vi "Obtain Queue Registry.vi"(8 "error in (no error)":errorcluster) -> (0 "error out":errorcluster, 2 "Queue Registry":map{string, refnum<queue>}(c390), 3 "Queue Registry Notifier":refnum<notifier>)   [LabVIEW 2021]
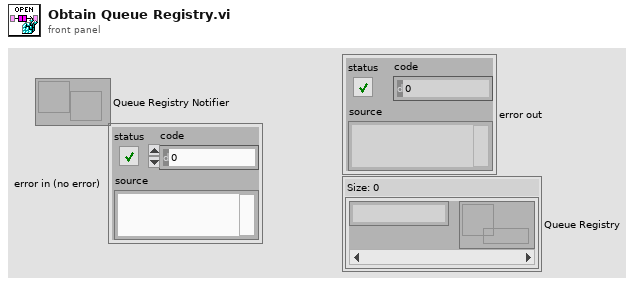
[diagram p1: front panel]
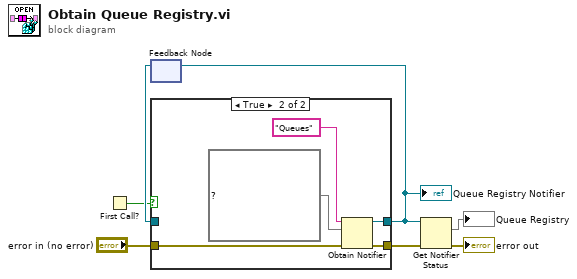
[diagram p0: block diagram]
diagram:
  n1 = First Call?() -> (First Call?: T/F=w6:bool)
  n2 = feedback #1() -> (w7:refnum<notifier>)  [unwired: 1 in]
  n3 = case shown="True" w6 {
    tunnel: [w9 w13] -> w4
    tunnel: w7 -> [w9 _]
    tunnel: [w8 w11] -> w3
    tunnel: "error in (no error)" -> [w8 w10]
    frame False {
    }
    frame True {
      n4 = Obtain Notifier(name (unnamed)="Queues", notification data type=map{string, refnum<queue>} {} ("map"), error in (no error)=w10) -> (notifier out=w13:refnum<notifier>, error out=w11:errorcluster)  [unwired: 1 in, 1 out]
    }
  }
  "Queue Registry Notifier" <- w4
  n5 = feedback-in #1(w4) -> ()
  n6 = Get Notifier Status(notifier=w4, error in (no error)=w3) -> (current notification=→"Queue Registry":map{string, refnum<queue>}, error out=→"error out":errorcluster)  [unwired: 3 out]
